vi "UDP Refresh Packet Sizes.vi"(8 "error in (no error)":errorcluster, 10 "UDP UI References in":T2, 11 "node References":T1) -> (0 "error out":errorcluster, 2 "UDP UI References out":T2, 3 "node References out":T1)   [LabVIEW 2015, in "E2E Tag Exchange editor node.lvclass"]
uses:
  E2E Tag Exchange editor node.lvclass
  UDP UI References.ctl
  object references.ctl
  <vilib>/NI/DCAF/Tag Editor Core/Configuration Editor/Classes/Engine Parent/Engine Parent Editor Node.lvclass
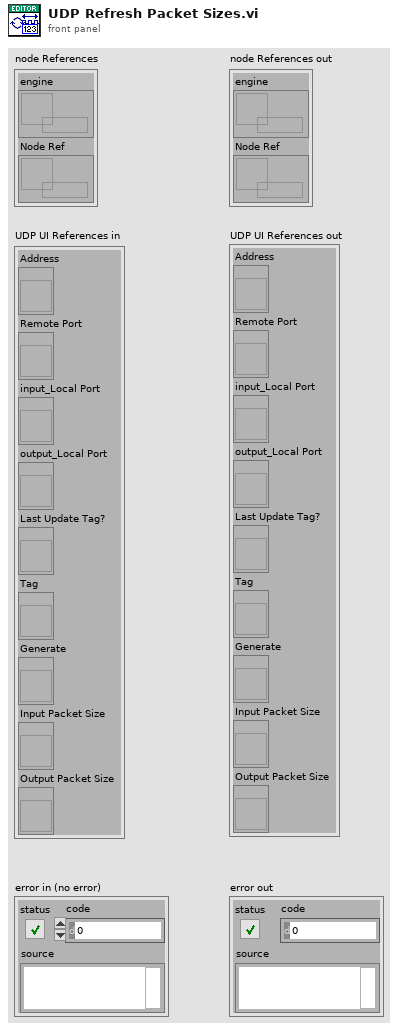
[diagram p1: front panel]
types:
  T1 = typedef "E2E Tag Exchange editor node.lvclass/object references.ctl" = cluster{"engine":refnum<data-value>, "Node Ref":refnum<data-value>}
  T2 = typedef "E2E Tag Exchange editor node.lvclass/UDP UI References.ctl" = cluster{"Address":refnum<vi>, "Remote Port":refnum<vi>, "input_Local Port":refnum<vi>, "output_Local Port":refnum<vi>, "Last Update Tag?":refnum<vi>, "Tag":refnum<vi>, "Generate":refnum<vi>, "Input Packet Size":refnum<vi>, "Output Packet Size":refnum<vi>}
  T3 = typedef "TBM channel.lvclass/data tables.ctl" = cluster{"input data":T4, "processing parameter":T4, "processing result":T4, "output data":T4}
  T4 = typedef "tag bus.lvlib/dictionary table pair.ctl" = cluster{"data dictionary":refnum<class "data dictionary.lvclass">, "data table":T5}
  T5 = typedef "tag bus.lvlib/data table.lvlib/data table.ctl" = cluster{"Double":dbl[], "Single":sgl[], "I64":i64[], "I32":i32[], "I16":i16[], "I8":i8[], "U64":u64[], "U32":u32[], "U16":u16[], "U8":u8[], "Boolean":bool[], "String":string[], "Array of Double":cluster{"DBL Array":dbl[]}[], "Array of Single":cluster{"SGL Array":sgl[]}[], "Array of I64":cluster{"I64 Array":i64[]}[], "Array of I32":cluster{"I32 Array":i32[]}[], "Array of I16":cluster{"I16 Array":i16[]}[], "Array of I8":cluster{"I8 Array":i8[]}[], "Array of U64":cluster{"U64 Array":u64[]}[], "Array of U32":cluster{"U32 Array":u32[]}[], "Array of U16":cluster{"U16 Array":u16[]}[], "Array of U8":cluster{"U8 Array":u8[]}[], "Array of Boolean":cluster{"Boolean Array":bool[]}[], "Array of String":cluster{"String Array":string[]}[]}
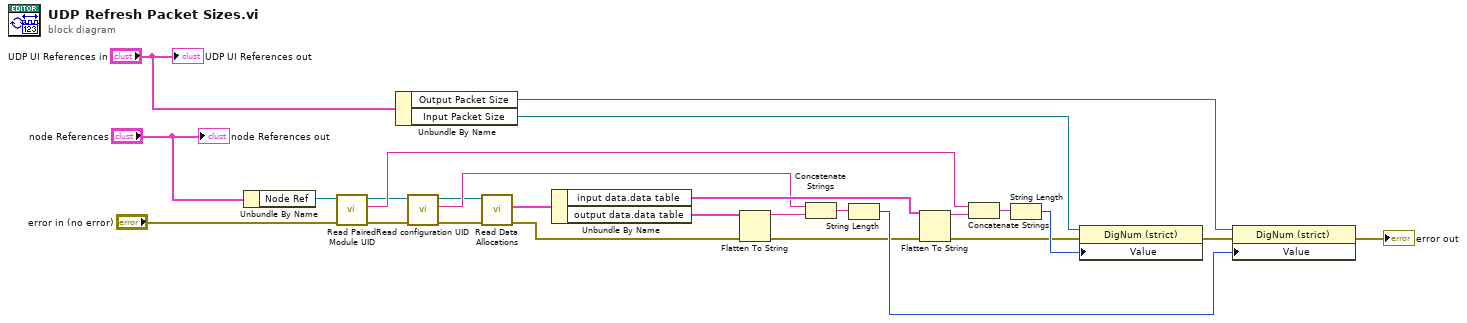
[diagram p0: block diagram]
diagram:
  n1 = Unbundle By Name("node References") -> ("Node Ref"=w26:refnum<data-value>)
  n2 = call "Read Paired Module UID.vi"("error in (no error)"="error in (no error)", "E2E editor node in"=w26) -> ("error out"=w9:errorcluster, "Paired Module UID"=w12:string, "E2E editor node out"=w6:refnum<data-value>)  [unwired: 7 in]
  n3 = Unbundle By Name("UDP UI References in") -> ("Output Packet Size"=w23:refnum<vi>, "Input Packet Size"=w20:refnum<vi>)
  n4 = call "Read configuration UID.vi"("error in (no error)"=w9, "E2E editor node in"=w6) -> ("error out"=w16:errorcluster, "Module UID"=w8:string, "E2E editor node out"=w7:refnum<data-value>)  [unwired: 7 in]
  n5 = call "Read Data Allocations.vi"("error in (no error)"=w16, "E2E editor node in"=w7) -> ("error out"=w17:errorcluster, "data allocations"=w15:T3)  [unwired: 7 in, 1 out]
  n6 = Unbundle By Name(w15) -> ("input data.data table"=w11:T5, "output data.data table"=w4:T5)
  n7 = Flatten To String(anything=w4, error in (no error)=w17) -> (data string=w3:string, error out=w10:errorcluster)  [unwired: 2 in, 1 out]
  n8 = Concatenate Strings(w8, w3) -> (w13:string)
  n9 = String Length(string=w13) -> (length=w22:i32)
  n10 = Flatten To String(anything=w11, error in (no error)=w10) -> (data string=w5:string, error out=w18:errorcluster)  [unwired: 2 in, 1 out]
  n11 = Concatenate Strings(w12, w5) -> (w14:string)
  n12 = String Length(string=w14) -> (length=w19:i32)
  n13 = property class="DigNum (strict)"(reference=w20, error in=w18, "Value"=w19) -> (error out=w21:errorcluster)  [unwired: 1 out]
  n14 = property class="DigNum (strict)"(reference=w23, error in=w21, "Value"=w22) -> (error out=→"error out":errorcluster)  [unwired: 1 out]
  "UDP UI References out" <- "UDP UI References in"
  "node References out" <- "node References"
